vi "trace_idxGlobal.vi"(0 "traces_spectrum":cluster{"idx":u32}[](array[cluster]), 1 "traces_interferogram":T2(array[cluster]), 5 "trace idx":u32, 7 "dataType":T1, 11 "error in (no error)":errorcluster) -> (4 "global trace idx":u32, 15 "error out":errorcluster)   [LabVIEW 2010, in "OSA.lvclass"]
uses:
  OSA.lvclass
  typeDef/acq_dataType.ctl
  OSA20X_misc.lvlib
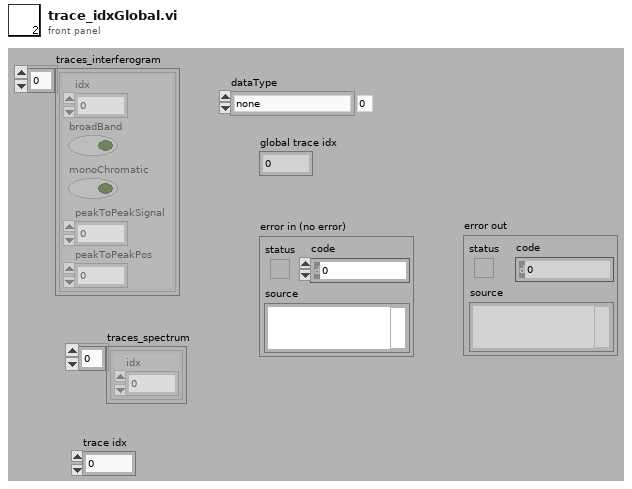
[diagram p1: front panel]
types:
  T1 = typedef "OSA.lvclass/acq_dataType.ctl" = enum16{"none", "interferogram", "spectrum"}
  T2 = cluster{"idx":u32, "broadBand":bool, "monoChromatic":bool, "peakToPeakSignal":dbl, "peakToPeakPos":dbl}[]
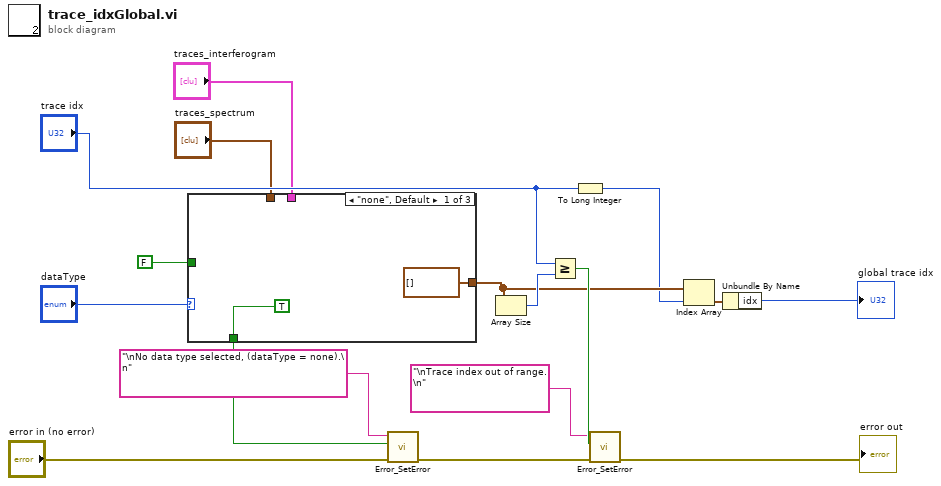
[diagram p0: block diagram]
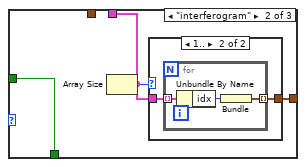
[diagram p2: hidden frame]
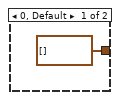
[diagram p3: hidden frame]
diagram:
  n1 = case shown="\"none\", Default" "dataType" {
    tunnel: "traces_interferogram" -> [_ w22 _]
    tunnel: "traces_spectrum" -> [_ _ w31]
    tunnel: [cluster{"idx":u32}[] [] ("traces") w21 w31] -> w14
    tunnel: [TRUE ("x >= y?") w20 w30] -> w4
    tunnel: FALSE ("x >= y?") -> [_ w20 w30]
    frame "none", Default {
    }
    frame "interferogram" {
      n2 = Array Size(array=w22) -> (size(s)=w23:i32)
      n3 = case shown="1.." w23 {
        tunnel: w22 -> [_ w26]
        tunnel: [cluster{"idx":u32}[] [] w25] -> w21
        frame 0, Default {
        }
        frame 1.. {
          n4 = for {
            tunnel: w26 -> [w29] mode=indexing
            tunnel: [w27] -> w25 mode=indexing
            n5 = Unbundle By Name(w29) -> ("idx"=w28:u32)
            n6 = Bundle("idx"=w28) -> (w27:cluster{"idx":u32})  [unwired: 1 in]
          }
        }
      }
    }
    frame "spectrum" {
    }
  }
  n7 = call "Error_SetError.vi"("error in"="error in (no error)", "status (true)"=w4, "source(\"\")"="\nNo data type selected, (dataType = none).\n" ("source(\"\")")) -> ("error out"=w2:errorcluster)  [unwired: 4 in]
  n8 = Array Size(array=w14) -> (size(s)=w15:i32)
  n9 = Greater Or Equal?(x="trace idx", y=w15) -> (x >= y?=w17:bool)
  n10 = To Long Integer(number="trace idx") -> (32bit integer=w7:i32)
  n11 = call "Error_SetError.vi"("error in"=w2, "status (true)"=w17, "source(\"\")"="\nTrace index out of range.\n" ("source(\"\")")) -> ("error out"=→"error out":errorcluster)  [unwired: 4 in]
  n12 = Index Array(array=w14, index=w7) -> (element=w13:cluster{"idx":u32})
  n13 = Unbundle By Name(w13) -> ("idx"=→"global trace idx":u32)
